vi "Chamber controller Sept 2017.vi"() -> ()   [LabVIEW 2014]
uses:
  <vilib>/Instr/_visa.llb/VISA Configure Serial Port (Instr).vi
  Environmental Chamber LabVIEW and Instruments/Drivers and Software/Keithley 2100 Series/Public/Configure/Configure 2 Wire Resistance.vi
  <vilib>/Utility/file.llb/Write To Spreadsheet File (string).vi
  <vilib>/Utility/file.llb/Read From Spreadsheet File (string).vi
  Environmental Chamber LabVIEW and Instruments/Drivers and Software/LabVIEW 8.2 Drivers/keithley_24xx/Keithley 24XX/Public/Data/Read (Single Point).vi
  Environmental Chamber LabVIEW and Instruments/Drivers and Software/keithley_24xx/Keithley 24XX/Keithley 24XX.lvlib
  Environmental Chamber LabVIEW and Instruments/Drivers and Software/keithley_6430/Keithley 6430/Keithley 6430.lvlib
  Environmental Chamber LabVIEW and Instruments/Drivers and Software/Keithley 2100 Series/Keithley 2100 Series.lvlib
panel:
  in  "Enable Auto Range (T:Enable)":bool=TRUE
  in  "K2420-range":dbl=1.0 format="%#_13g"
  in  "K2420 Applied Voltage (V)":dbl=0.1
  out "Hz":dbl format="%#.7f"
  in  "Gate time (s)":enum16{"0.1", "1.0 ", "10"}(ring)=enum."1.0 "
  out "QCM plot":T1(graph)
  in  "K6340 Bias (V)":dbl min=-30.0 max=30.0
  out "K-2420 2":cluster{"Resistance":sgl}(graph)
  in  "points":i32=10
  in  "average points?":bool
  in  "Pressure parameters cluster":T2={"valve % open"=0.0, "Desired pressure"=0.0, "Vapor sccm"=0.0, "Gas sccm"=0.0, "Valve mode"=enum."% Open", "Pressure Mode"=enum."Abs. pressure", "analyte partial pressure"=23.8, "Turbo pump\nauto on"=TRUE, "Valve position (%)"=0.0, "read pressure"=0.0, "read vapor flow"=0.0, "read gas flow"=0.0} caption="Pressure settings" {"read gas flow" format="%#_3g"; "read vapor flow" format="%#_3g"; "read pressure" format="%#_7f"; "Valve position (%)" format="%#_3g"; "analyte partial pressure" min=0.0 max=100.0 step=5.0; "Gas sccm" min=0 max=200 step=5; "Vapor sccm" min=0 max=200 step=5; "Desired pressure" min=0.0 max=760.0 step=5.0; "valve % open" min=0.0 max=100.0 step=5.0 format="%#_2f"}
  out "pressure chart":cluster{"pressure":dbl}(graph)
  out "arduino qcm stack plot":T3(graph)
  out "saving data?":bool
  in  "Data logging settings":T4={"Save during sequence only"=TRUE, "Save now"=FALSE, "sec between points"=0.0, "Current data file path"=path "", "Save sample/gas names"={"QCM1"="", "QCM2"="", "QCM3"="", "QCM4"="", "QCM5"="NOT WORKING", "QCM6"="", "SRS"="bareAu", "K-2420"="", "K-6430"="", "K-2100"="", "Gas"="NOT WORKING", "Vapor"="H2O"}, "add notes to file"=FALSE} {"sec between points" min=0.0 max=30.0 format="%#_13g"}
  in  "Sequence cluster":T5={"Save sequence"=FALSE, "Clear sequence"=FALSE, "Import sequence file"=FALSE, "Run Sequence"=FALSE, "Stop program when sequence ends"=TRUE, "User-defined\nsequence"=[], "Sequence end time"="", "Sequence\npreview"=[], "Current\nstep"=0, "Display"=0, "Sequence length (hrs)"=0.0} caption="Pressure settings" {"Display" items=["pressure", "gas flow", "vapor flow", "bias"]}
  out "J-KEM temp chart":dbl(graph)
  out "State date/time":string caption="Start time"
  out "K-2100 (Ohm)":cluster{"Measurement":dbl}(graph) caption="K-2100"
  in  "Stop":bool
  in  "Clear all charts":bool
  out "O2 sensor output":dbl[](array[numeric]) caption="atm\nTorr"
  in  "rapidox O2 Sensor":bool
  in  "setnag O2 Pump":bool
  in  "Baud Rate 2":i32(ring)=2 items=["2400", "4800", "9600", "19200", "38400", "57600", "115200"]
  in  "Com Port":i32(ring) items=["Com 1", "Com 2", "Com 3", "Com 4", "Com 5", "Com 6", "COM 7", "COM 8", "COM 9", "COM 10", "COM 11", "COM 12", "com 13", "COM 14"]
  in  "Com Port 2":i32(ring) items=["Com 1", "Com 2", "Com 3", "Com 4", "Com 5", "Com 6", "COM 7", "COM 8", "COM 9", "COM 10", "COM 11", "COM 12", "com 13", "COM 14"]
  out "Waveform Chart":cluster{dbl}(graph)
  out "O2 Concentration (PPM)":dbl
  out "Waveform Chart 6":cluster{dbl}(graph)
  # "SRS"
  # "Currently Unused"
  # "100%"
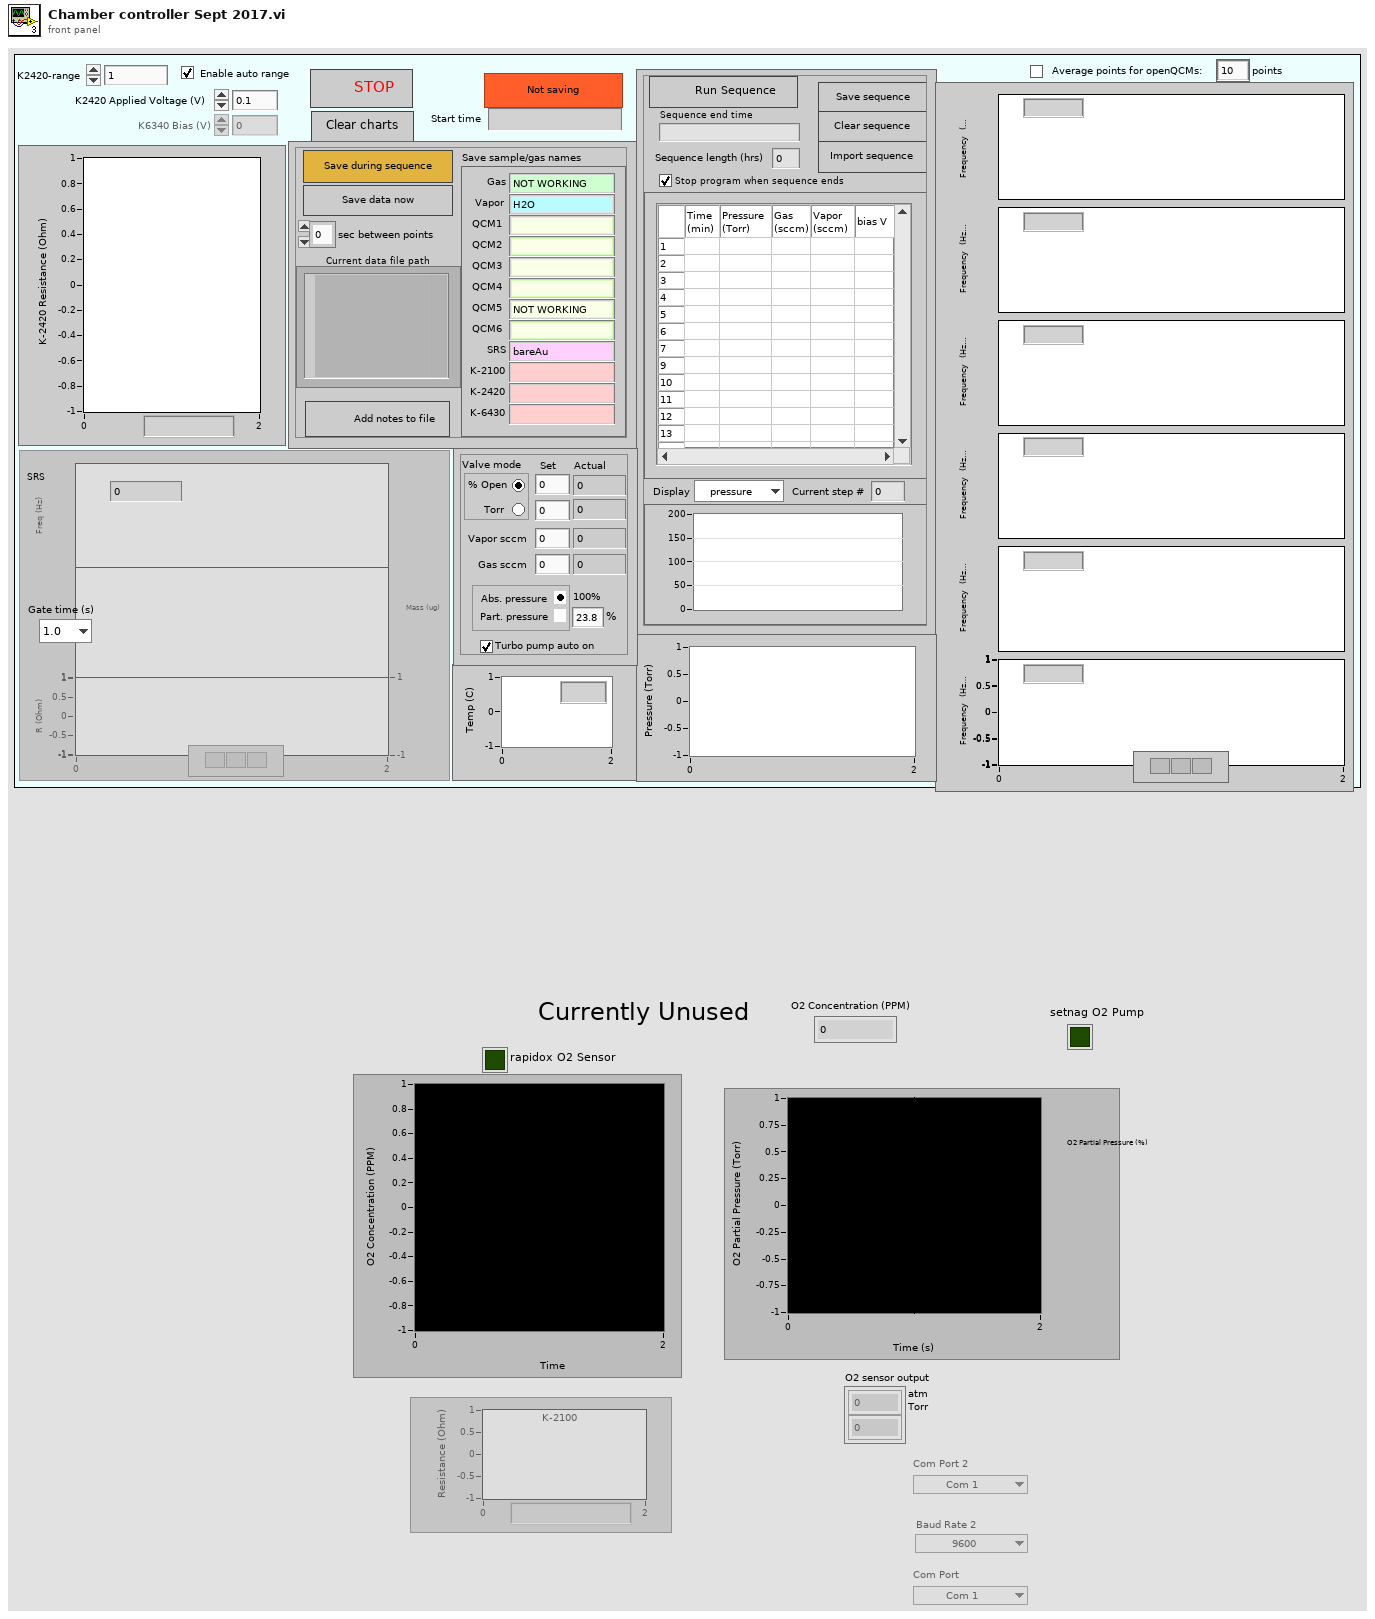
[diagram p1: front panel]
types:
  T1 = cluster{"Frequency out":dbl, "Numeric Control":dbl, "Resistance out":dbl}
  T2 = cluster{"valve % open":dbl, "Desired pressure":dbl, "Vapor sccm":sgl, "Gas sccm":sgl, "Valve mode":enum32{"% Open", "Torr "}, "Pressure Mode":enum32{"Abs. pressure", " Part. pressure"}, "analyte partial pressure":dbl, "Turbo pump\nauto on":bool, "Valve position (%)":dbl, "read pressure":dbl, "read vapor flow":dbl, "read gas flow":dbl}
  T3 = cluster{"mean":dbl, "mean":dbl, "mean":dbl, "mean":dbl, "mean":dbl, "mean":dbl}
  T4 = cluster{"Save during sequence only":bool, "Save now":bool, "sec between points":dbl, "Current data file path":path, "Save sample/gas names":cluster{"QCM1":string, "QCM2":string, "QCM3":string, "QCM4":string, "QCM5":string, "QCM6":string, "SRS":string, "K-2420":string, "K-6430":string, "K-2100":string, "Gas":string, "Vapor":string}, "add notes to file":bool}
  T5 = cluster{"Save sequence":bool, "Clear sequence":bool, "Import sequence file":bool, "Run Sequence":bool, "Stop program when sequence ends":bool, "User-defined\nsequence":string[][], "Sequence end time":string, "Sequence\npreview":cluster{dbl[], dbl[]}[], "Current\nstep":i32, "Display":u16, "Sequence length (hrs)":dbl}
  T6 = cluster{"Keithley 6430":bool, "J-KEM":bool, "Keithley 2420":bool, "Keithley 2100":bool, "SRS QCM":bool, "Pressure control":bool, "Arduino":bool}
  T7 = cluster{"Arduino 1":refnum<visa-resource-name>, "Arduino 2":refnum<visa-resource-name>, "Arduino 3":refnum<visa-resource-name>, "Arduino 4":refnum<visa-resource-name>, "Arduino 5":refnum<visa-resource-name>, "Arduino 6":refnum<visa-resource-name>}
  T8 = enum8{"Enabled", "Disabled", "Disabled and Grayed Out"}
  T9 = enum16{"open", "open or create", "create or replace", "create", "open (read only)"}
  T10 = enum16{"no parity", "odd parity", "even parity", "mark parity", "space parity"}
  T11 = cluster{"mean":dbl, "mean":dbl, "mean":dbl, "mean":dbl, "mean":dbl, "mean":dbl}[]
  T12 = cluster{"Frequency out":dbl, "Numeric Control":dbl, "Resistance out":dbl}[]
  T13 = cluster{"String":string, "String":string, "String":string}
  T14 = cluster{bool, "task out":refnum<k21>, "error out":errorcluster, "task out":refnum<k21>, "error out":errorcluster, "turbo pump":refnum<visa-resource-name>, "error out":errorcluster}
  T15 = cluster{bool, "task out":refnum<k21>, "error out":errorcluster, "task out":refnum<k21>, "error out":errorcluster, "VISA resource name out":refnum<visa-resource-name>, "error out":errorcluster}
  T16 = cluster{bool, "VISA resource name":refnum<visa-resource-name>, "error out":errorcluster}
  T17 = cluster{bool, "VISA resource name out":refnum<visa-resource-name>, "error out":errorcluster}
  T18 = cluster{"VISA resource name out":refnum<visa-resource-name>, "error out":errorcluster, "VISA resource name out":refnum<visa-resource-name>, "error out":errorcluster, "VISA resource name out":refnum<visa-resource-name>, "error out":errorcluster, "VISA resource name out":refnum<visa-resource-name>, "error out":errorcluster, "VISA resource name out":refnum<visa-resource-name>, "error out":errorcluster, "VISA resource name out 2":refnum<visa-resource-name>, "error out 2":errorcluster}
  T19 = cluster{"Boolean":bool, "VISA resource name out":refnum<visa-resource-name>, "error out":errorcluster}
  T20 = cluster{bool, "VISA out":refnum<visa-resource-name>, "error out":errorcluster}
  T21 = cluster{"Boolean":bool, "VISA out":refnum<visa-resource-name>, "error out":errorcluster}
  T22 = cluster{"Numeric Control":dbl, "Cluster":cluster{"Numeric Control":dbl}, "String":string, "error out":errorcluster}
  T23 = cluster{bool, "Com Port":i32, "Numeric Control out":dbl}
  T24 = cluster{"Arduino address":refnum<visa-resource-name>, "error in (no error)":errorcluster, "Arduino address 2":refnum<visa-resource-name>, "error in (no error) 2":errorcluster, "Arduino address 3":refnum<visa-resource-name>, "error in (no error) 3":errorcluster, "Arduino address 4":refnum<visa-resource-name>, "error in (no error) 4":errorcluster, "Arduino address 5":refnum<visa-resource-name>, "error in (no error) 5":errorcluster, "Arduino address 6":refnum<visa-resource-name>, "error in (no error) 6":errorcluster}
  T25 = cluster{"String":string, "String":string, "String":string, "String":string, "String":string, "String":string}
  T26 = cluster{"valve % open":dbl, "Desired pressure":dbl, "Vapor sccm":sgl, "Gas sccm":sgl, "Valve mode":enum32{"% Open", "Torr "}, "Pressure Mode":enum32{"Abs. pressure", " Part. pressure"}, "analyte partial pressure":dbl}
  T27 = cluster{"User-defined\nsequence":string[][], "Present (s)":dbl, "current  step # in":i32, "sequence end time in":timestamp}
  T28 = cluster{"current  step # in":i32, "sequence end time in":timestamp, "Boolean":bool}
  T29 = cluster{"press/RH/gas/vapor":cluster{"pressure":string, "RH":string, "gas flow":string, "vapor flow":string}, "Cluster":cluster{"Valve position (%)":dbl, "read pressure":dbl, "read vapor flow":dbl, "read gas flow":dbl}}
  T30 = cluster{"Boolean":bool, "task out":refnum<k21>, "error out":errorcluster, "task out":refnum<k21>, "error out":errorcluster, "VISA resource name out":refnum<visa-resource-name>, "error out":errorcluster}
  T31 = cluster{"String":dbl, "String":dbl, "String":dbl, "String":dbl, "String":dbl, "String":dbl}
  T32 = cluster{"pressure":string, "RH":string, "gas flow":string, "vapor flow":string}
  T33 = cluster{"Valve position (%)":dbl, "read pressure":dbl, "read vapor flow":dbl, "read gas flow":dbl}
  T34 = cluster{"f":dbl, "f":dbl, "f":dbl, "f":dbl, "f":dbl}[]
  T35 = cluster{"QCM1":string, "QCM2":string, "QCM3":string, "QCM4":string, "QCM5":string, "QCM6":string, "SRS":string, "K-2420":string, "K-6430":string, "K-2100":string, "Gas":string, "Vapor":string}
  T36 = cluster{"String data out":string, string, string, string}
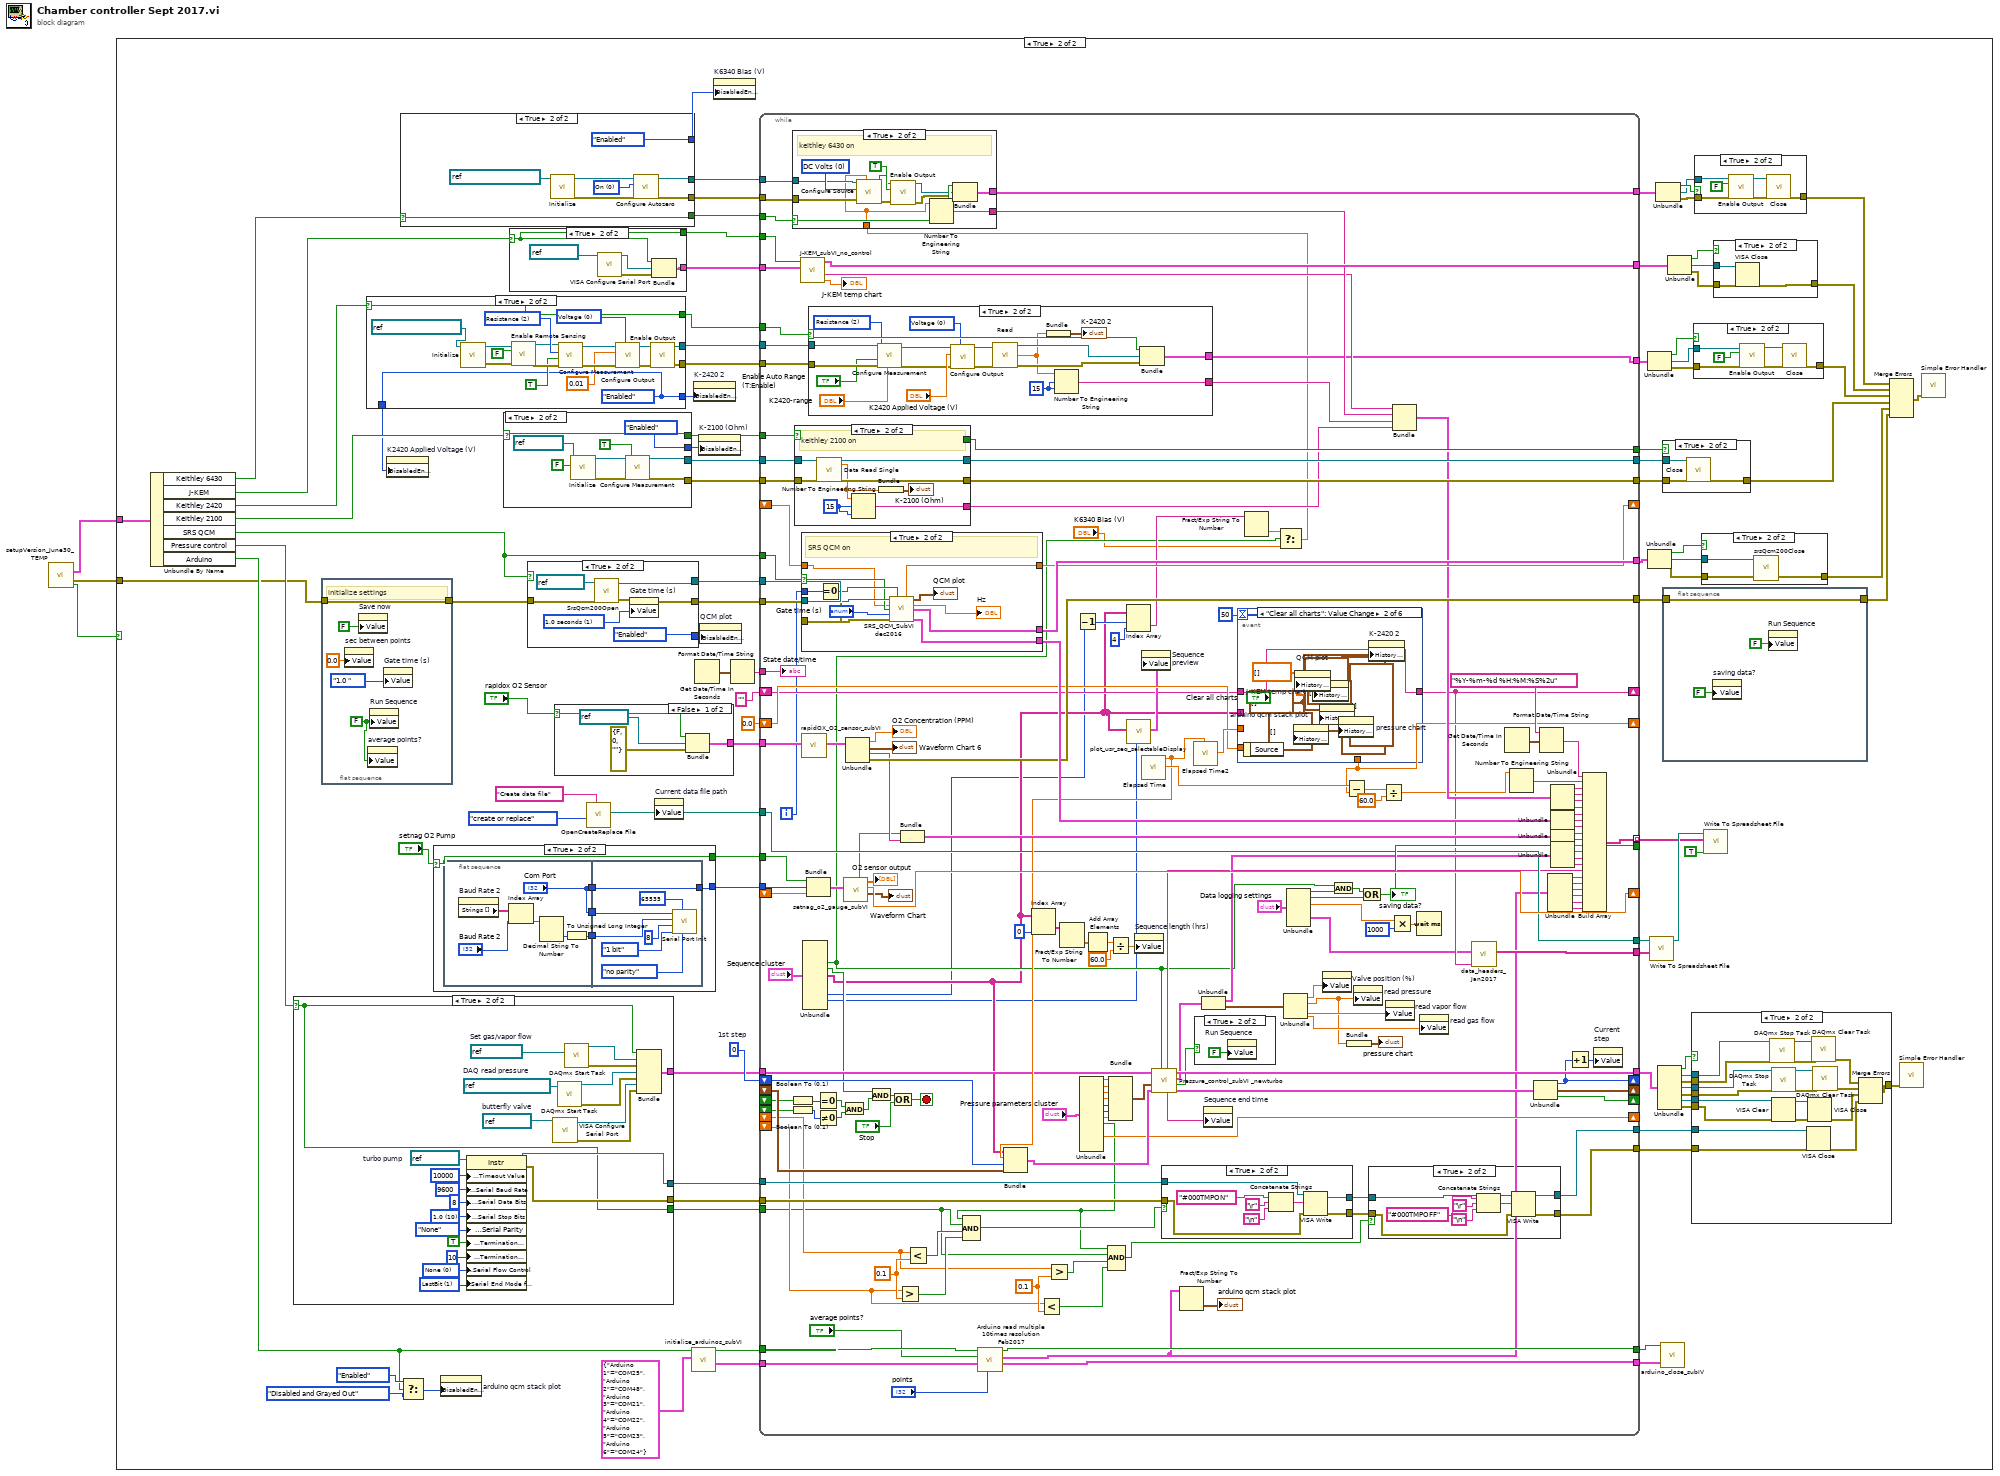
[diagram p0: block diagram]
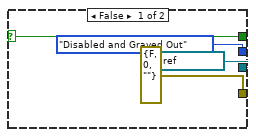
[diagram p4: hidden frame]
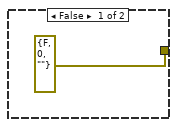
[diagram p5: hidden frame]
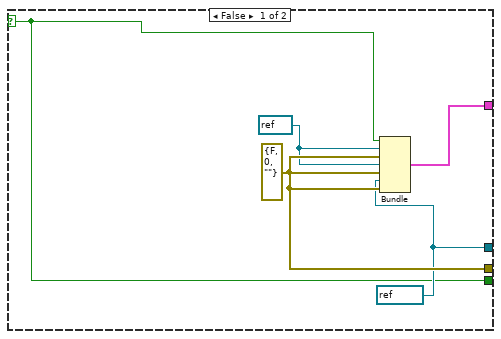
[diagram p6: hidden frame]
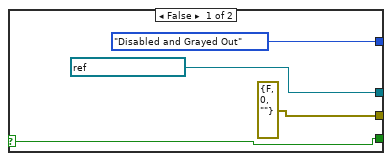
[diagram p8: hidden frame]
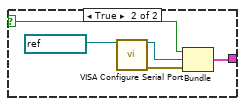
[diagram p9: hidden frame]
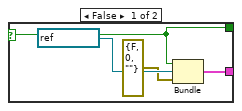
[diagram p11: hidden frame]
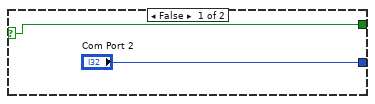
[diagram p12: hidden frame]
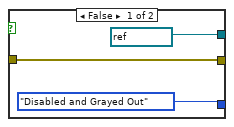
[diagram p14: hidden frame]
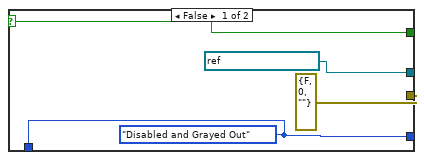
[diagram p16: hidden frame]
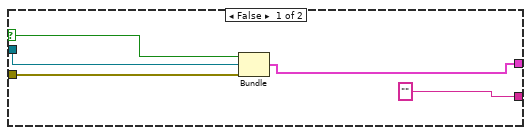
[diagram p17: hidden frame]
diagram:
  n1 = call "setupVersion_June30_TEMP.vi"() -> ("Instruments on/off"=w1:T6, "error IO"=w2:errorcluster, "OK"=w3:bool)  [unwired: 13 in]
  n2 = case shown="True" w3 {
    tunnel: w2 -> [_ w23]
    tunnel: w1 -> [_ w33]
    frame False {
    }
    frame True {
      w39 = 0  # 1st step
      n3 = Unbundle By Name(w33) -> ("Keithley 6430"=w32:bool, "J-KEM"=w31:bool, "Keithley 2420"=w30:bool, "Keithley 2100"=w29:bool, "SRS QCM"=w28:bool, "Pressure control"=w27:bool, "Arduino"=w26:bool)
      n4 = case shown="True" w27 {
        selector: w27 -> [w145 w150]
        tunnel: [w149 w151] -> w21
        tunnel: [w148 w153] -> w13
        tunnel: [w146 w152] -> w14
        tunnel: [w145 w150] -> w12
        frame False {
          w146 = refnum<visa-resource-name> refnum ("turbo pump")
          w147 = refnum<k21> refnum ("task out")
          w148 = errorcluster {"status"=FALSE, "code"=0, "source"=""} ("error out")
          n5 = Bundle(w145, "task out"=w147, "error out"=w148, "task out"=w147, "error out"=w148, "turbo pump"=w146, "error out"=w148) -> (w149:T14)  [unwired: 1 in]
        }
        frame True {
          w157 = u16 1 items=["None", "LastBit", "TermChar"] ("Serial Settings:Serial End Mode for Reads")
          w155 = u16 0 items=["None", "XON/XOFF", "RTS/CTS", "XON/XOFF & RTS/CTS", "DTR/DSR", "XON/XOFF & DTR/DSR"] ("flow control (0:none)")
          w158 = u16 10 items=["1.0"=10, "1.5"=15, "2.0"=20] ("stop bits (10: 1 bit)")
          w154 = refnum<visa-resource-name> "COM7"  # turbo pump
          w170 = refnum<visa-resource-name> "COM5"  # butterfly valve
          w171 = refnum<k21> "Setflow"  # Set gas/vapor flow
          w172 = refnum<k21> "AllDaqReadings"  # DAQ read pressure
          n6 = property class="Instr"(reference=w154, "General Settings:Timeout Value"=u32 10000 ("timeout (10sec)"), "Serial Settings:Serial Baud Rate"=u32 9600 ("baud rate (9600)"), "Serial Settings:Serial Data Bits"=u16 8 ("data bits (8)"), "Serial Settings:Serial Stop Bits"=w158, "Serial Settings:Serial Parity"=enum16{"None", "Odd", "Even", "Mark", "Space"}."None" ("parity (0:none)"), "Message Based Settings:Termination Character Enable"=TRUE ("Enable Termination\nChar (T)"), "Message Based Settings:Termination Character"=u8 10 ("termination char\n(0xA = '\\n' = LF)"), "Serial Settings:Serial Flow Control"=w155, "Serial Settings:Serial End Mode for Reads"=w157) -> (reference out=w152:refnum<visa-resource-name>, error out=w153:errorcluster)  [unwired: 1 in]
          n7 = call-poly "VISA Configure Serial Port"("VISA resource name"=w170) -> ("VISA resource name out"=w165:refnum<visa-resource-name>, "error out"=w164:errorcluster)  [unwired: 13 in]
          n8 = call <vilib>:"DAQmx Start Task.vi"("task/channels in"=w172) -> ("task out"=w167:refnum<k21>, "error out"=w166:errorcluster)  [unwired: 13 in]
          n9 = call <vilib>:"DAQmx Start Task.vi"("task/channels in"=w171) -> ("task out"=w169:refnum<k21>, "error out"=w168:errorcluster)  [unwired: 13 in]
          n10 = Bundle(w150, "task out"=w169, "error out"=w168, "task out"=w167, "error out"=w166, "VISA resource name out"=w165, "error out"=w164) -> (w151:T15)  [unwired: 1 in]
        }
      }
      n11 = flat-sequence {
        tunnel: [w101] -> w22
        tunnel: w23 -> [w101]
        frame #0 {
          w100 = FALSE ("Value")
          # "initialize settings"
          n12 = property on="sec between points" class="DigNum (strict)"("Value"=0.0) -> ()  [unwired: 2 in, 2 out]
          n13 = property on="Save now" class="Bool (strict)"("Value"=FALSE) -> ()  [unwired: 2 in, 2 out]
          n14 = property on="average points?" class="Bool (strict)"("Value"=w100) -> ()  [unwired: 2 in, 2 out]
          n15 = property on="Run Sequence" class="Bool (strict)"("Value"=w100) -> ()  [unwired: 2 in, 2 out]
          n16 = property on="Gate time (s)" class="Enum (strict)"("Value"=enum16{"0.1", "1.0 ", "10"}."1.0 " ("Gate time (sec)")) -> ()  [unwired: 2 in, 2 out]
        }
      }
      n17 = case shown="True" w30 {
        selector: w30 -> [w256 w261]
        tunnel: [refnum<visa-resource-name> "GPIB1::24::INSTR" ("VISA resource name") w269] -> w97
        tunnel: [errorcluster {"status"=FALSE, "code"=0, "source"=""} ("error out") w264] -> w96
        tunnel: [w255 w260] -> w6
        tunnel: [w256 w261] -> w55
        tunnel: [w255 w260] -> w4
        frame False {
          w255 = T8."Disabled and Grayed Out" ("Disabled")
        }
        frame True {
          w260 = T8."Enabled" ("Disabled")
          w270 = u16 0 items=["Voltage", "Current"] ("Source Mode  (0: Voltage)")
          w275 = u16 2 items=["Volts", "Current", "Resistance"] ("Function (0: Volts)")
          n18 = call "Initialize.vi"("VISA resource name"=refnum<visa-resource-name> "GPIB1::24::INSTR") -> ("error out"=w265:errorcluster, "VISA resource name out"=w268:refnum<visa-resource-name>)  [unwired: 9 in]
          n19 = call "Enable Remote Sensing.vi"("error in (no error)"=w265, "Enable Remote Sensing (T: Enable)"=FALSE ("4-wire?"), "VISA resource name"=w268) -> ("error out"=w266:errorcluster, "VISA resource name out"=w267:refnum<visa-resource-name>)  [unwired: 7 in]
          n20 = call "Configure Measurement.vi"("error in (no error)"=w266, "Enable Auto Range (T:Enable)"=TRUE, "Function (0: Volts)"=w275, "VISA resource name"=w267) -> ("error out"=w274:errorcluster, "VISA resource name out"=w273:refnum<visa-resource-name>)  [unwired: 6 in]
          n21 = call "Configure Output.vi"("Source Mode  (0: Voltage)"=w270, "error in (no error)"=w274, "Output Level (0)"=0.01 ("K2420 Applied Voltage (V) 2"), "VISA resource name"=w273) -> ("error out"=w272:errorcluster, "VISA resource name out"=w271:refnum<visa-resource-name>)  [unwired: 6 in]
          n22 = call "Enable Output.vi"("error in (no error)"=w272, "VISA resource name"=w271) -> ("error out"=w264:errorcluster, "VISA resource name out"=w269:refnum<visa-resource-name>)  [unwired: 8 in]
        }
      }
      n23 = property on="K2420 Applied Voltage (V)" class="DigNum (strict)"("DisabledEnum"=w4) -> ()  [unwired: 2 in, 2 out]
      n24 = case shown="True" w32 {
        selector: w32 -> [w180 w190]
        tunnel: [refnum<visa-resource-name> "GPIB0::29::INSTR" ("VISA resource name") w185] -> w66
        tunnel: [errorcluster {"status"=FALSE, "code"=0, "source"=""} ("error out") w184] -> w65
        tunnel: [T8."Disabled and Grayed Out" ("Disabled") T8."Enabled" ("Disabled")] -> w5
        tunnel: [w180 w190] -> w54
        frame False {
        }
        frame True {
          w189 = u16 0 items=["On", "Off", "Once"] ("Autozero  (0: On)")
          n25 = call "Initialize.vi"("VISA resource name"=refnum<visa-resource-name> "GPIB2::19::INSTR") -> ("error out"=w188:errorcluster, "VISA resource name out"=w187:refnum<visa-resource-name>)  [unwired: 4 in, 5 out]
          n26 = call "Configure Autozero.vi"("error in (no error)"=w188, "Autozero  (0: On)"=w189, "VISA resource name"=w187) -> ("error out"=w184:errorcluster, "VISA resource name out"=w185:refnum<visa-resource-name>)  [unwired: 7 in]
        }
      }
      n27 = Select(t=T8."Enabled" ("Disabled"), s=w26, f=T8."Disabled and Grayed Out" ("Disabled")) -> (s? t:f=w7:T8)
      n28 = case shown="True" "setnag O2 Pump" {
        selector: "setnag O2 Pump" -> [w214 w216]
        tunnel: ["Com Port 2" w217] -> w93
        tunnel: [w214 w216] -> w44
        frame False {
        }
        frame True {
          n29 = flat-sequence {
            tunnel: ["Com Port"] -> w220
            tunnel: [w222] -> w219
            tunnel: ["Com Port"] -> w218
            tunnel: w220 -> [w228]
            tunnel: w219 -> [w227]
            tunnel: w218 -> [w229]
            tunnel: [w229] -> w217
            frame #0 {
              n30 = property on="Baud Rate 2" class="Ring (strict)"() -> ("Strings []"=w224:string[])  [unwired: 2 in, 2 out]
              n31 = Index Array(array=w224, index="Baud Rate 2") -> (element=w225:string)
              n32 = Decimal String To Number(string=w225) -> (number=w223:i32)  [unwired: 2 in, 1 out]
              n33 = To Unsigned Long Integer(number=w223) -> (unsigned 32bit integer=w222:u32)
            }
            frame #1 {
              n34 = call <vilib>:"Serial Port Init.vi"("parity"=T10."no parity", "buffer size"=u16 65535, "stop bits"=enum16{"1 bit", "1.5 bits", "2 bits"}."1 bit", "data bits"=u16 8, "baud rate"=w227, "port number"=w228) -> ()  [unwired: 1 in, 1 out]
            }
          }
        }
      }
      n35 = property on="arduino qcm stack plot" class="WFChart (strict)"("DisabledEnum"=w7) -> ()  [unwired: 2 in, 2 out]
      n36 = case shown="True" w29 {
        selector: w29 -> [w113 w118]
        tunnel: [refnum<visa-resource-name> "K-2100" ("VISA resource name out") w121] -> w53
        tunnel: [errorcluster {"status"=FALSE, "code"=0, "source"=""} ("error out") w120] -> w52
        tunnel: [w113 w118] -> w51
        tunnel: [T8."Disabled and Grayed Out" ("Disabled") T8."Enabled" ("Disabled")] -> w46
        frame False {
        }
        frame True {
          n37 = call "Initialize.vi"("VISA resource name"=refnum<visa-resource-name> "K-2100", "Reset? (T: Reset)"=FALSE) -> ("VISA resource name out"=w122:refnum<visa-resource-name>, "error out"=w119:errorcluster)  [unwired: 16 in]
          n38 = call-poly "Configure Measurement.vi"("VISA resource name"=w122, "error in (no error)"=w119, "Auto Range? (T: Auto)"=TRUE) -> ("VISA resource name out"=w121:refnum<visa-resource-name>, "error out"=w120:errorcluster)  [unwired: 15 in]
        }
      }
      n39 = case shown="True" w31 {
        selector: w31 -> [w205 w210]
        tunnel: [w206 w211] -> w82
        tunnel: [w205 w210] -> w76
        frame False {
          n40 = Bundle(w205, "VISA resource name"=refnum<visa-resource-name> "COM3", "error out"=errorcluster {"status"=FALSE, "code"=0, "source"=""}) -> (w206:T16)  [unwired: 1 in]
        }
        frame True {
          n41 = call-poly "VISA Configure Serial Port"("VISA resource name"=refnum<visa-resource-name> "COM3") -> ("VISA resource name out"=w212:refnum<visa-resource-name>, "error out"=w209:errorcluster)  [unwired: 13 in]
          n42 = Bundle(w210, "VISA resource name out"=w212, "error out"=w209) -> (w211:T17)  [unwired: 1 in]
        }
      }
      n43 = case shown="True" w28 {
        tunnel: [refnum<visa-resource-name> "COM6" ("VISA in") w244] -> w95
        tunnel: [w239 w241] -> w94
        tunnel: w22 -> [w239 w246]
        tunnel: [T8."Disabled and Grayed Out" ("Disabled") T8."Enabled" ("Disabled")] -> w61
        frame False {
        }
        frame True {
          w243 = u16 1 items=["0.1 seconds", "1.0 seconds", "10.0 seconds"] ("Gate time")
          n44 = call "SrsQcm200Open.vi"("error in"=w246, "VISA in"=refnum<visa-resource-name> "COM6") -> ("error out"=w242:errorcluster, "VISA out"=w244:refnum<visa-resource-name>)  [unwired: 3 in]
          n45 = property on="Gate time (s)" class="Enum (strict)"(error in=w242, "Value"=w243) -> (error out=w241:errorcluster)  [unwired: 1 in, 1 out]
        }
      }
      n46 = case shown="False" "rapidox O2 Sensor" {
        selector: "rapidox O2 Sensor" -> [w192 w197]
        tunnel: [w193 w198] -> w72
        frame False {
          n47 = Bundle(w192, "VISA resource name"=refnum<visa-resource-name> "COM7", "error out"=errorcluster {"status"=FALSE, "code"=0, "source"=""}) -> (w193:T16)  [unwired: 1 in]
        }
        frame True {
          n48 = call-poly "VISA Configure Serial Port"("VISA resource name"=refnum<visa-resource-name> "COM7") -> ("VISA resource name out"=w199:refnum<visa-resource-name>, "error out"=w196:errorcluster)  [unwired: 13 in]
          n49 = Bundle(w197, "VISA resource name out"=w199, "error out"=w196) -> (w198:T17)  [unwired: 1 in]
        }
      }
      n50 = call "OpenCreateReplace File.vi"("prompt"="Create data file", "function (open:0)"=T9."create or replace") -> ("new file path"=w9:path)  [unwired: 6 in, 3 out]
      n51 = property on="Current data file path" class="Path"("Value"=w9) -> ()  [unwired: 2 in, 2 out]
      n52 = call "initialize_arduinos_subVI.vi"("arduino 1-6 addresses"=T7 {"Arduino 1"="COM25", "Arduino 2"="COM48", "Arduino 3"="COM21", "Arduino 4"="COM22", "Arduino 5"="COM23", "Arduino 6"="COM24"} ("Arduino COMs"), "arduinos on?"=w26) -> ("arduino addresses/errors"=w40:T18, "arduinos on/off"=w59:bool)  [unwired: 8 in]
      n53 = property on="K-2420 2" class="WFChart (strict)"("DisabledEnum"=w6) -> ()  [unwired: 2 in, 2 out]
      n54 = Get Date/Time In Seconds() -> (seconds since 1Jan1904=w99:timestamp)
      n55 = property on="K-2100 (Ohm)" class="WFChart (strict)"("DisabledEnum"=w46) -> ()  [unwired: 2 in, 2 out]
      n56 = property on="QCM plot" class="WFChart (strict)"("DisabledEnum"=w61) -> ()  [unwired: 2 in, 2 out]
      n57 = property on="K6340 Bias (V)" class="DigNum (strict)"("DisabledEnum"=w5) -> ()  [unwired: 2 in, 2 out]
      n58 = Format Date/Time String(seconds (now)=w99) -> (date/time string=w43:string)  [unwired: 2 in]
      n59 = while {
        shift-right: [w454] -> _
        shift-left: _ -> [w395]
        tunnel: [w442] -> w60 mode=indexing if=w416
        tunnel: w55 -> [w315]
        tunnel: w97 -> [w317]
        tunnel: w96 -> [w316]
        tunnel: w95 -> [w453]
        tunnel: w94 -> [w452]
        tunnel: w28 -> [w451]
        tunnel: w44 -> [w397]
        tunnel: w93 -> [w398]
        tunnel: [w312] -> w90
        tunnel: [w450] -> w86
        tunnel: w82 -> [w449]
        tunnel: [w448] -> w81
        tunnel: w76 -> [w447]
        tunnel: w72 -> [w405]
        tunnel: [w401] -> w25
        tunnel: [w346] -> w71
        tunnel: w9 -> [w346]
        shift-right: [w440] -> _
        shift-left: _ -> [w441]
        tunnel: w66 -> [w446]
        tunnel: w65 -> [w445]
        tunnel: [w444] -> w64
        tunnel: [w416] -> _
        tunnel: w59 -> [w291]
        tunnel: w40 -> [w292]
        tunnel: [w289] -> w57
        tunnel: [w288] -> w58
        tunnel: [w293] -> w56
        tunnel: w54 -> [w428]
        tunnel: w53 -> [w415]
        tunnel: w52 -> [w414]
        tunnel: w51 -> [w413]
        tunnel: [w412] -> w50
        tunnel: [w411] -> w49
        tunnel: [w410] -> w48
        shift-right: [w389] -> _
        shift-left: 0.0 ("Elapsed Time (s)") -> [w390]
        tunnel: w43 -> [w380]
        tunnel: w21 -> [w340]
        shift-right: [w343] -> _
        shift-left: w39 -> [w357]
        shift-right: [w362] -> _
        shift-left: _ -> [w360]
        shift-right: [w361] -> _
        shift-left: _ -> [w359]
        shift-left: _ -> [w358]
        tunnel: [w355] -> w38
        tunnel: w14 -> [w335]
        tunnel: w13 -> [w334]
        tunnel: w12 -> [w324]
        tunnel: [w329] -> w11
        tunnel: [w330] -> w10
        shift-right: [w339] -> _
        shift-left: _ -> [w326]
        shift-left: _ -> [w325]
        shift-right: [w295] -> _
        shift-left: "" ("notes to add") -> [w309]
        i -> [w296]
        stop <- w418 stop-if-true
        w328 = 0.1 ("y")
        w338 = 0.1 ("y")
        n60 = Boolean To (0,1)(Boolean=w359) -> (0, 1=w426:i16)
        n61 = Boolean To (0,1)(Boolean=w358) -> (0, 1=w425:i16)
        n62 = case shown="True" w413 {
          selector: w413 -> [w501 w506]
          tunnel: [w502 w513] -> w411
          tunnel: [w503 w512] -> w410
          tunnel: w415 -> [w502 w511]
          tunnel: w414 -> [w503 w510]
          tunnel: ["" w508] -> w399
          tunnel: [w501 w506] -> w412
          frame False {
            # "keithley 2100 off"
          }
          frame True {
            w505 = i16 15 ("width (-)")
            # "keithley 2100 on"
            n63 = call "Data Read Single.vi"("VISA resource name"=w511, "error in (no error)"=w510) -> ("VISA resource name out"=w513:refnum<visa-resource-name>, "Measurement"=w509:dbl, "error out"=w512:errorcluster)  [unwired: 15 in]
            n64 = Number To Engineering String ("elapsed time (min)")(2:w505, 3:w505, 4:w509) -> (0:w508:string)  [unwired: 1 in]
            n65 = Bundle("Measurement"=w509) -> (→"K-2100 (Ohm)":cluster{"Measurement":dbl})  [unwired: 1 in]
          }
        }
        n66 = call "J-KEM_subVI_no_control.vi"("Address in"=w449, "J-KEM on?"=w447) -> ("Temp (C)"=→"J-KEM temp chart":dbl, "String data out"=w388:string, "Address out"=w448:T19)  [unwired: 6 in, 1 out]
        n67 = case "SRS QCM" shown="True" w451 {
          selector: w451 -> [w548 w558]
          tunnel: w453 -> [w551 w560]
          tunnel: w452 -> [w550 w562]
          tunnel: [w549 w555] -> w450
          tunnel: w441 -> [w546 w556]
          tunnel: [w546 w557] -> w440
          tunnel: [T13 {"String"="", "String"="", "String"=""} ("M,F,MR output cluster") w554] -> w433
          tunnel: w296 -> [_ w563]
          frame False {
            # "SRS QCM off"
            n68 = Bundle(w548, "VISA out"=w551, "error out"=w550) -> (w549:T20)  [unwired: 1 in]
          }
          frame True {
            # "SRS QCM on"
            n69 = Equal To 0?(x=w563) -> (x = 0?=w559:bool)
            n70 = call "SRS_QCM_SubVI  dec2016.vi"("VISA Refnum in"=w560, "first iteration?"=w559, "Frequency  in"=w556, "SRS on?"=w558, "Gate time"="Gate time (s)", "error in (no error)"=w562) -> ("Frequency out 2"=w557:dbl, "freq, mass, MR"=→"QCM plot":T1, "Frequency out"=→"Hz":dbl, "address out"=w555:T21, "M,F,MR output cluster"=w554:T13)  [unwired: 2 in, 3 out]
          }
        }
        n71 = call "rapidOX_O2_sensor_subVI.vi"("rapid ox info in"=w405) -> ("rapidox info out"=w404:T22)  [unwired: 10 in]
        n72 = Unbundle("Sequence cluster") -> ("Run Sequence"=w302:bool, "Stop program when sequence ends"=w301:bool, "User-defined\nsequence"=w300:string[][], "Current\nstep"=w299:i32, "Display"=w298:u16)  [unwired: 6 out]
        n73 = Bundle(w397, "Com Port"=w398, "Numeric Control out"=w395) -> (w396:T23)  [unwired: 1 in]
        n74 = case shown="True" w315 {
          selector: w315 -> [w460 w479]
          tunnel: ["" w478] -> w311
          tunnel: [w457 w477] -> w312
          tunnel: w317 -> [w459 w467]
          tunnel: w316 -> [w458 w465]
          frame False {
            n75 = Bundle(w460, "VISA resource name out"=w459, "error out"=w458) -> (w457:T17)  [unwired: 1 in]
          }
          frame True {
            w461 = u16 2 items=["Volts", "Current", "Resistance"] ("Function (0: Volts)")
            w471 = u16 0 items=["Voltage", "Current"] ("Source Mode  (0: Voltage)")
            w472 = i16 15 ("width (-)")
            n76 = call "Configure Measurement.vi"("Manual Range (1.0)"="K2420-range", "error in (no error)"=w465, "Enable Auto Range (T:Enable)"="Enable Auto Range (T:Enable)", "Function (0: Volts)"=w461, "VISA resource name"=w467) -> ("error out"=w464:errorcluster, "VISA resource name out"=w466:refnum<visa-resource-name>)  [unwired: 5 in]
            n77 = call "Configure Output.vi"("Source Mode  (0: Voltage)"=w471, "error in (no error)"=w464, "Output Level (0)"="K2420 Applied Voltage (V)", "VISA resource name"=w466) -> ("error out"=w469:errorcluster, "VISA resource name out"=w470:refnum<visa-resource-name>)  [unwired: 6 in]
            n78 = call-poly "Read.vi"("VISA resource name"=w470, "error in (no error)"=w469) -> ("VISA resource name out"=w475:refnum<visa-resource-name>, "Resistance"=w473:sgl, "error out"=w474:errorcluster)  [unwired: 7 in, 4 out]
            n79 = Bundle("Resistance"=w473) -> (→"K-2420 2":cluster{"Resistance":sgl})  [unwired: 1 in]
            n80 = Number To Engineering String(2:w472, 3:w472, 4:w473) -> (0:w478:string)  [unwired: 1 in]
            n81 = Bundle(w479, "VISA resource name out"=w475, "error out"=w474) -> (w477:T17)  [unwired: 1 in]
          }
        }
        n82 = Equal To 0?(x=w426) -> (x = 0?=w423:bool)
        n83 = Not Equal To 0?(x=w425) -> (x != 0?=w424:bool)
        n84 = And(x=w423, y=w424) -> (x .and. y?=w417:bool)
        n85 = call "setnag_o2_gauge_subVI.vi"("setnag info in"=w396) -> ("Cluster"=→"Waveform Chart":cluster{"Numeric Control":dbl}, "Numeric Control out"=w454:dbl, "Array"=→"O2 sensor output":dbl[], "String"=w344:string)  [unwired: 7 in]
        n86 = Unbundle(w404) -> ("Numeric Control"=→"O2 Concentration (PPM)":dbl, "Cluster"=→"Waveform Chart 6":cluster{"Numeric Control":dbl}, "String"=w379:string, "error out"=w401:errorcluster)
        n87 = And(x=w301, y=w417) -> (x .and. y?=w393:bool)
        n88 = Or(x=w393, y="Stop") -> (x .or. y?=w418:bool)
        n89 = Greater?(x=w325, y=w338) -> (0:w337:bool)
        n90 = Bundle("String"=w344, "String"=w379) -> (w378:cluster{"String":string, "String":string})  [unwired: 1 in]
        n91 = Less?(x=w326, y=w338) -> (x < y?=w336:bool)
        n92 = call "Arduino read multiple 10times resolution Feb2017.vi"("# of points to average"="points", "arduino addresses in"=w292, "average points?"="average points?", "arduinos on?"=w291) -> ("arduino addresses out"=w288:T24, "freq out"=w285:T25, "arduinos on"=w289:bool)  [unwired: 4 in]
        n93 = Index Array(array=w300, index (col)=0 ("disabled index (col)")) -> (element=w307:string[])  [unwired: 1 in]
        n94 = Less?(x=w325, y=w328) -> (x < y?=w322:bool)
        n95 = Greater?(x=w326, y=w328) -> (0:w323:bool)
        n96 = Fract/Exp String To Number(string=w307) -> (number=w306:dbl[])  [unwired: 3 in, 1 out]
        n97 = Decrement(x=w299) -> (x-1=w319:i32)
        n98 = Unbundle("Pressure parameters cluster") -> ("valve % open"=w369:dbl, "Desired pressure"=w370:dbl, "Vapor sccm"=w371:sgl, "Gas sccm"=w372:sgl, "Valve mode"=w373:enum32{"% Open", "Torr "}, "Pressure Mode"=w374:enum32{"Abs. pressure", " Part. pressure"}, "analyte partial pressure"=w375:dbl, "Turbo pump\nauto on"=w327:bool, "read pressure"=w339:dbl)  [unwired: 3 out]
        n99 = Compound Arithmetic op=AND(w327, w324, w336, w337) -> (w333:bool)
        n100 = Add Array Elements(numeric array=w306) -> (sum=w305:dbl)
        n101 = Compound Arithmetic op=AND(w327, w324, w323, w322) -> (w321:bool)
        n102 = Divide(x=w305, y=60.0) -> (x/y=w303:dbl)
        n103 = Bundle("valve % open"=w369, "Desired pressure"=w370, "Vapor sccm"=w371, "Gas sccm"=w372, "Valve mode"=w373, "Pressure Mode"=w374, "analyte partial pressure"=w375) -> (w368:T26)  [unwired: 1 in]
        n104 = Index Array(array=w300, index (row)=w319, index (col)=4 ("disabled index (col)")) -> (element=w314:string)
        n105 = call "plot_usr_seq_selectableDisplay.vi"("Display"=w298, "User-defined sequence"=w300) -> ("Sequence Preview"=w318:cluster{dbl[], dbl[]}[])  [unwired: 9 in]
        n106 = property on="Sequence length (hrs)" class="DigNum (strict)"("Value"=w303) -> ()  [unwired: 2 in, 2 out]
        n107 = property on="Sequence\npreview" class="XYGraph (strict)"("Value"=w318) -> ()  [unwired: 2 in, 2 out]
        n108 = call "Elapsed Time"() -> ("Present (s)"=w364:dbl, "Elapsed Time (s)"=w407:dbl)  [unwired: 12 in, 6 out]
        n109 = Bundle("User-defined\nsequence"=w300, "Present (s)"=w364, "current  step # in"=w357, "sequence end time in"=w360) -> (w365:T27)  [unwired: 1 in]
        n110 = call "Pressure_control_subVI _newturbo.vi"("Run Sequence"=w302, "user sequence, present (s) in, current step in, seq time in"=w365, "pressure parameters in"=w368, "pressure control on?/daq IDs/errors"=w340) -> ("current step # out, shift register time out, seq button on?"=w363:T28, "sequence over? USE THIS TO REINITIALIZE RUN SEQUENCE BUTTON SO PROGRAM ENDS"=w354:bool, "save press/RH/gasflow/vaporflow - read valve position/pressure/vaporflow/gasflow"=w353:T29, "pressure control on?/daq IDs/errors out"=w355:T30, "sequence end date/time string"=w356:string, "pressure_setpoint"=w341:string)  [unwired: 2 in]
        n111 = case shown="True" w333 {
          tunnel: w335 -> [w491 w494]
          tunnel: w334 -> [w490 w495]
          tunnel: [w491 w493] -> w332
          tunnel: [w490 w492] -> w331
          frame False {
          }
          frame True {
            n112 = Concatenate Strings("#000TMPON" ("write buffer 2"), "\r", "\n") -> (w496:string)
            n113 = VISA Write(VISA resource name=w494, write buffer=w496, error in (no error)=w495) -> (VISA resource name out=w493:refnum<visa-resource-name>, error out=w492:errorcluster)  [unwired: 1 out]
          }
        }
        n114 = Fract/Exp String To Number(string=w285) -> (number=→"arduino qcm stack plot":T31)  [unwired: 3 in, 1 out]
        n115 = call "Elapsed Time2"("Set Start Time (s)"=w364) -> ("Elapsed Time (s)"=w391:dbl)  [unwired: 11 in, 7 out]
        n116 = case shown="True" w354 {
          frame False {
          }
          frame True {
            n117 = property on="Run Sequence" class="Bool (strict)"("Value"=FALSE ("Run Sequence")) -> ()  [unwired: 2 in, 2 out]
          }
        }
        n118 = Unbundle(w353) -> ("press/RH/gas/vapor"=w352:T32, "Cluster"=w351:T33)
        n119 = property on="Sequence end time" class="Str"("Value"=w356) -> ()  [unwired: 2 in, 2 out]
        n120 = event shown="[1] \"Clear all charts\": Value Change" {
          selector: _ -> [_ _ _ _ _ _]
          dyn-events: _ -> [_ _ _ _ _ _]
          timeout: 50 -> [_ _ _ _ _ _]
          tunnel: w300 -> [_ _ _ _ w526 _]
          tunnel: w391 -> [_ _ _ _ _ _]
          tunnel: w390 -> [w515 _ _ _ _ _]
          tunnel: [w515 _ _ _ _ _] -> w389
          tunnel: [w514 w518 w522 w523 w525 w527] -> w295
          tunnel: w309 -> [w514 w518 w521 w523 w525 w527]
          event Timeout {
            n121 = event-data() -> ()  [unwired: 1 in, 1 out]
          }
          event "Clear all charts": Value Change {
            (unwired) T34 [] ("History Data")
            w516 = cluster{dbl}[] [] ("History Data")
            (unwired) cluster{"Resistance":sgl}[] [] ("History Data")
            (unwired) cluster{dbl, "Resistance out":dbl}[] [] ("History Data")
            n122 = event-data() -> ()  [unwired: 1 in, 1 out]
            n123 = property on="Waveform Chart" class="WFChart (strict)"("History Data"=w516) -> ()  [unwired: 2 in, 2 out]
            n124 = property on="QCM plot" class="WFChart (strict)"("History Data"=T12 []) -> ()  [unwired: 2 in, 2 out]
            n125 = property on="J-KEM temp chart" class="WFChart (strict)"("History Data"=dbl[] []) -> ()  [unwired: 2 in, 2 out]
            n126 = property on="arduino qcm stack plot" class="WFChart (strict)"("History Data"=T11 []) -> ()  [unwired: 2 in, 2 out]
            n127 = property on="pressure chart" class="WFChart (strict)"("History Data"=w516) -> ()  [unwired: 2 in, 2 out]
            n128 = property on="K-2420 2" class="WFChart (strict)"("History Data"=w516) -> ()  [unwired: 2 in, 2 out]
          }
          event "Data logging settings.add notes to file": Value Change {
            n129 = event-data() -> ()  [unwired: 1 in, 1 out]
            n130 = call "notes_subVI.vi"("previous notes"=w521) -> ("notes to add"=w522:string)  [unwired: 14 in]
          }
          event "Sequence cluster.Clear sequence": Value Change {
            n131 = event-data() -> ()  [unwired: 1 in, 1 out]
            n132 = property on="User-defined\nsequence" class="Tbl (strict)"("Value"=string[][] []) -> ()  [unwired: 2 in, 2 out]
          }
          event "Sequence cluster.Save sequence": Value Change {
            n133 = event-data() -> ()  [unwired: 1 in, 1 out]
            n134 = call-poly <vilib>:"Write To Spreadsheet File.vi"("2D data"=w526) -> ()  [unwired: 7 in, 1 out]
          }
          event "Sequence cluster.Import sequence file": Value Change {
            n135 = event-data() -> ()  [unwired: 1 in, 1 out]
            n136 = call-poly <vilib>:"Read From Spreadsheet File.vi"() -> ("all rows"=w528:string[][])  [unwired: 7 in, 4 out]
            n137 = property on="User-defined\nsequence" class="Tbl (strict)"("Value"=w528) -> ()  [unwired: 2 in, 2 out]
          }
        }
        n138 = Fract/Exp String To Number(string=w314) -> (number=w313:dbl)  [unwired: 3 in, 1 out]
        n139 = Select(t=w313, s=w302, f="K6340 Bias (V)") -> (s? t:f=w277:dbl)
        n140 = case "Keithley 6430" shown="True" w428 {
          selector: w428 -> [w532 w545]
          tunnel: w446 -> [w531 w536]
          tunnel: w445 -> [w530 w537]
          tunnel: ["" w544] -> w400
          tunnel: [w529 w543] -> w444
          tunnel: w277 -> [_ w534]
          frame False {
            # "keithley 6430 off"
            n141 = Bundle(w532, "VISA resource name out"=w531, "error out"=w530) -> (w529:T17)  [unwired: 1 in]
          }
          frame True {
            w541 = u16 0 items=["DC Volts", "DC Current"] ("Source Function (0: DC Volts)")
            # "keithley 6430 on"
            n142 = call "Configure Source.vi"("V-Source Level [V]"=w534, "error in (no error)"=w537, "Source Function (0: DC Volts)"=w541, "VISA resource name"=w536) -> ("error out"=w538:errorcluster, "VISA resource name out"=w535:refnum<visa-resource-name>)  [unwired: 6 in]
            n143 = call "Enable Output.vi"("error in (no error)"=w538, "Enable Output (F:Off)"=TRUE ("Output (F:Off)"), "VISA resource name"=w535) -> ("error out"=w539:errorcluster, "VISA resource name out"=w540:refnum<visa-resource-name>)  [unwired: 7 out]
            n144 = Number To Engineering String(4:w534) -> (0:w544:string)  [unwired: 3 in]
            n145 = Bundle(w545, "VISA resource name out"=w540, "error out"=w539) -> (w543:T17)  [unwired: 1 in]
          }
        }
        n146 = Unbundle(w351) -> ("Valve position (%)"=w350:dbl, "read pressure"=w345:dbl, "read vapor flow"=w349:dbl, "read gas flow"=w348:dbl)
        n147 = Unbundle("Data logging settings") -> ("Save during sequence only"=w420:bool, "Save now"=w422:bool, "sec between points"=w409:dbl, "Save sample/gas names"=w294:T35)  [unwired: 2 out]
        n148 = property on="Valve position (%)" class="DigNum (strict)"("Value"=w350) -> ()  [unwired: 2 in, 2 out]
        n149 = And(x=w302, y=w420) -> (x .and. y?=w419:bool)
        n150 = Subtract(x=w407, y=w389) -> (x-y=w406:dbl)
        n151 = Bundle("read pressure"=w345) -> (→"pressure chart":cluster{"read pressure":dbl})  [unwired: 1 in]
        n152 = property on="read pressure" class="DigNum (strict)"("Value"=w345) -> ()  [unwired: 2 in, 2 out]
        n153 = Or(x=w419, y=w422) -> (x .or. y?=w416:bool)
        "saving data?" <- w416
        n154 = case shown="True" w321 {
          tunnel: w332 -> [w481 w484]
          tunnel: w331 -> [w480 w485]
          tunnel: [w481 w483] -> w329
          tunnel: [w480 w482] -> w330
          frame False {
          }
          frame True {
            n155 = Concatenate Strings("#000TMPOFF" ("write buffer 2"), "\r", "\n") -> (w486:string)
            n156 = VISA Write(VISA resource name=w484, write buffer=w486, error in (no error)=w485) -> (VISA resource name out=w483:refnum<visa-resource-name>, error out=w482:errorcluster)  [unwired: 1 out]
          }
        }
        n157 = Divide(x=w406, y=60.0) -> (x/y=w381:dbl)
        n158 = property on="read vapor flow" class="DigNum (strict)"("Value"=w349) -> ()  [unwired: 2 in, 2 out]
        n159 = Multiply(x=w409, y=u32 1000 ("x")) -> (x*y=w437:dbl)
        n160 = Bundle("String data out"=w388, w400, w311, w399) -> (w394:T36)  [unwired: 1 in]
        n161 = Wait (ms)(milliseconds to wait=w437) -> ()  [unwired: 1 out]
        n162 = property on="read gas flow" class="DigNum (strict)"("Value"=w348) -> ()  [unwired: 2 in, 2 out]
        n163 = call "data_headers_Jan2017.vi"("Experiment Notes"=w295, "Sample names"=w294) -> ("data headers"=w293:string[])  [unwired: 9 in]
        n164 = Get Date/Time In Seconds() -> (seconds since 1Jan1904=w455:timestamp)
        n165 = Number To Engineering String ("elapsed time (min)")(4:w381) -> (0:w386:string)  [unwired: 3 in]
        n166 = Unbundle(w363) -> ("current  step # in"=w343:i32, "sequence end time in"=w362:timestamp, "Boolean"=w361:bool)
        n167 = Format Date/Time String(time format string (%c)="%Y-%m-%d %H:%M:%S%2u", seconds (now)=w455) -> (date/time string=w434:string)  [unwired: 1 in]
        n168 = Unbundle(w285) -> ("String"=w284:string, "String"=w283:string, "String"=w282:string, "String"=w281:string, "String"=w280:string, "String"=w279:string)
        n169 = Unbundle(w394) -> ("String data out"=w385:string, w384:string, w383:string, w382:string)
        n170 = Unbundle(w433) -> ("String"=w387:string, "String"=w436:string, "String"=w435:string)
        n171 = Unbundle(w378) -> ("String"=w377:string, "String"=w376:string)
        n172 = Unbundle(w352) -> ("pressure"=w432:string, "RH"=w431:string, "gas flow"=w430:string, "vapor flow"=w429:string)
        n173 = Increment(x=w343) -> (x+1=w342:i32)
        n174 = Build Array(w434, w386, w385, w384, w383, w382, w387, w436, w435, w377, w376, w432, w431, w430, w429, w341, w284, w283, w282, w281, w280, w279) -> (w442:string[])
        n175 = property on="Current\nstep" class="DigNum (strict)"("Value"=w342) -> ()  [unwired: 2 in, 2 out]
        "State date/time" <- w380
      }
      n176 = Unbundle(w90) -> (w89:bool, "VISA resource name out"=w88:refnum<visa-resource-name>, "error out"=w87:errorcluster)
      n177 = Unbundle(w86) -> ("Boolean"=w85:bool, "VISA out"=w84:refnum<visa-resource-name>, "error out"=w83:errorcluster)
      n178 = call-poly <vilib>:"Write To Spreadsheet File.vi"("1D data"=w56, "file path (dialog if empty)"=w71) -> ("new file path (Not A Path if cancelled)"=w75:path)  [unwired: 6 in]
      n179 = Unbundle(w64) -> (w69:bool, "VISA resource name out"=w68:refnum<visa-resource-name>, "error out"=w67:errorcluster)
      n180 = Unbundle(w38) -> ("Boolean"=w37:bool, "task out"=w20:refnum<k21>, "error out"=w19:errorcluster, "task out"=w18:refnum<k21>, "error out"=w17:errorcluster, "VISA resource name out"=w16:refnum<visa-resource-name>, "error out"=w15:errorcluster)
      n181 = call "arduino_close_subIV.vi"("arduino 1-6 addresses and errors out"=w58, "arduinos on?"=w57) -> ()  [unwired: 10 in]
      n182 = case shown="True" w50 {
        tunnel: w49 -> [_ w111]
        tunnel: w48 -> [w108 w110]
        tunnel: [w108 w109] -> w47
        frame False {
        }
        frame True {
          n183 = call "Close.vi"("VISA resource name"=w111, "error in (no error)"=w110) -> ("error out"=w109:errorcluster)  [unwired: 17 in]
        }
      }
      n184 = flat-sequence {
        tunnel: w25 -> [w107]
        tunnel: [w107] -> w24
        frame #0 {
          n185 = property on="saving data?" class="Bool (strict)"("Value"=FALSE ("saving data?")) -> ()  [unwired: 2 in, 2 out]
          n186 = property on="Run Sequence" class="Bool (strict)"("Value"=FALSE ("saving data?")) -> ()  [unwired: 2 in, 2 out]
        }
      }
      n187 = Unbundle(w81) -> ("Boolean"=w80:bool, "VISA resource name out"=w79:refnum<visa-resource-name>, "error out"=w78:errorcluster)
      n188 = case shown="True" w37 {
        tunnel: [errorcluster {"status"=FALSE, "code"=0, "source"=""} ("error out") w136] -> w42
        tunnel: w20 -> [_ w135]
        tunnel: w19 -> [_ w134]
        tunnel: w18 -> [_ w133]
        tunnel: w17 -> [_ w130]
        tunnel: w16 -> [_ w131]
        tunnel: w15 -> [_ w132]
        tunnel: w11 -> [_ w127]
        tunnel: w10 -> [_ w126]
        frame False {
        }
        frame True {
          n189 = call <vilib>:"DAQmx Stop Task.vi"("task/channels in"=w135, "error in"=w134) -> ("task out"=w142:refnum<k21>, "error out"=w141:errorcluster)  [unwired: 12 in]
          n190 = call <vilib>:"DAQmx Stop Task.vi"("task/channels in"=w133, "error in"=w130) -> ("task out"=w143:refnum<k21>, "error out"=w144:errorcluster)  [unwired: 12 in]
          n191 = VISA Clear(VISA resource name=w131, error in (no error)=w132) -> (VISA resource name out=w140:refnum<visa-resource-name>, error out=w139:errorcluster)
          n192 = VISA Close(VISA resource name=w127, error in (no error)=w126) -> (error out=w128:errorcluster)
          n193 = VISA Close(VISA resource name=w140, error in (no error)=w139) -> (error out=w129:errorcluster)
          n194 = call <vilib>:"DAQmx Clear Task.vi"("task in"=w142, "error in"=w141) -> ("error out"=w138:errorcluster)  [unwired: 13 in]
          n195 = call <vilib>:"DAQmx Clear Task.vi"("task in"=w143, "error in"=w144) -> ("error out"=w137:errorcluster)  [unwired: 13 in]
          n196 = Merge Errors(w138, w137, w129, w128) -> (w136:errorcluster)
        }
      }
      n197 = case shown="True" w89 {
        tunnel: w88 -> [_ w251]
        tunnel: w87 -> [w248 w250]
        tunnel: [w248 w249] -> w91
        frame False {
        }
        frame True {
          n198 = call "Enable Output.vi"("error in (no error)"=w250, "Enable Output (T: Enable)"=FALSE, "VISA resource name"=w251) -> ("error out"=w252:errorcluster, "VISA resource name out"=w254:refnum<visa-resource-name>)  [unwired: 7 in]
          n199 = call "Close.vi"("error in (no error)"=w252, "VISA resource name"=w254) -> ("error out"=w249:errorcluster)  [unwired: 9 in]
        }
      }
      n200 = case shown="True" w69 {
        tunnel: w68 -> [_ w175]
        tunnel: w67 -> [w173 w174]
        tunnel: [w173 w176] -> w63
        frame False {
        }
        frame True {
          n201 = call "Enable Output.vi"("error in (no error)"=w174, "Enable Output (F:Off)"=FALSE ("Output (F:Off)"), "VISA resource name"=w175) -> ("error out"=w177:errorcluster, "VISA resource name out"=w178:refnum<visa-resource-name>)  [unwired: 7 out]
          n202 = call "Close.vi"("error in (no error)"=w177, "VISA resource name"=w178) -> ("error out"=w176:errorcluster)  [unwired: 9 out]
        }
      }
      n203 = case shown="True" w85 {
        tunnel: w83 -> [w234 w237]
        tunnel: [w234 w236] -> w92
        tunnel: w84 -> [_ w235]
        frame False {
        }
        frame True {
          n204 = call "srsQcm200Close.vi"("error in"=w237, "Visa in"=w235) -> ("error out"=w236:errorcluster)  [unwired: 3 in]
        }
      }
      n205 = call-poly <vilib>:"Write To Spreadsheet File.vi"("append to file? (new file:F)"=TRUE, "2D data"=w60, "file path (dialog if empty)"=w75) -> ()  [unwired: 5 in, 1 out]
      n206 = case shown="True" w80 {
        tunnel: w79 -> [_ w204]
        tunnel: w78 -> [w201 w203]
        tunnel: [w201 w202] -> w77
        frame False {
        }
        frame True {
          n207 = VISA Close(VISA resource name=w204, error in (no error)=w203) -> (error out=w202:errorcluster)
        }
      }
      n208 = Merge Errors(w63, w77, w91, w47, w92, w24) -> (w98:errorcluster)
      n209 = call <vilib>:"Simple Error Handler.vi"("error in (no error)"=w42) -> ()  [unwired: 4 in, 5 out]
      n210 = call <vilib>:"Simple Error Handler.vi"("error in (no error)"=w98) -> ()  [unwired: 4 in, 5 out]
    }
  }
